vi "Trim Colon from NS.vi"(1 "String in":string) -> (0 "String out":string)   [LabVIEW 2018, in "Path and String Processing.lvlib"]
uses:
  Path and String Processing.lvlib
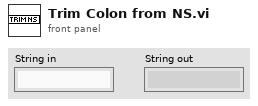
[diagram p1: front panel]
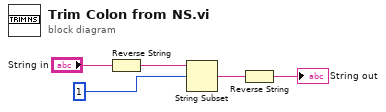
[diagram p0: block diagram]
diagram:
  n1 = Reverse String(1:"String in") -> (0:w5:string)
  n2 = String Subset(string=w5, offset (0)=1) -> (substring=w3:string)  [unwired: 1 in]
  n3 = Reverse String(1:w3) -> (0:→"String out":string)
